vi "rt-Voltage - Continuous Output.vi"() -> ()   [LabVIEW 2019]
doc: "This example demonstrates how to continuously re-generate analog output data from a buffer in your computer's memory.\n\nRefer to your device documentation for pinouts and hardware capabilities."
uses:
  <vilib>/Utility/error.llb/DialogType.ctl
  <vilib>/DAQmx/write.llb/DAQmx Write (Analog 1D Wfm NChan NSamp).vi
  <vilib>/DAQmx/create/channels.llb/DAQmx Create Channel (AO-Voltage-Basic).vi
  <vilib>/DAQmx/configure/timing.llb/DAQmx Timing (Sample Clock).vi
  <vilib>/DAQmx/configure/trigger.llb/DAQmx Start Trigger (Digital Edge).vi
  <vilib>/DAQmx/configure/trigger.llb/DAQmx Start Trigger (Time).vi
  <vilib>/DAQmx/configure/trigger.llb/DAQmx Start Trigger (Analog Edge).vi
  <vilib>/DAQmx/miscellaneous.llb/DAQmx Fill In Error Info.vi
  <resource>/objmgr/daqmx.rc
  <vilib>/measure/NI_MABase.lvlib
panel:
  in  "Trigger Type":T1(tab)
  in  "Digital Start Trigger Edge":i32(ring)=10280 caption="Edge" items=["Rising"=10280, "Falling"=10171]
  in  "Digital Start Trigger Source":tag="/Dev1/PFI0" caption="Source"
  in  "Digital Pause Trigger Pause When":i32(ring)=10192 caption="Pause When" items=["High"=10192, "Low"=10214]
  in  "Digital Pause Trigger Source":tag="/Dev1/PFI0" caption="Source"
  in  "Analog Start Trigger Level":dbl caption="Level" format="%0.2f"
  in  "Analog Start Trigger Hysteresis":dbl caption="Hysteresis" format="%.2f"
  in  "Analog Start Trigger Slope":i32(ring)=10280 caption="Slope" items=["Rising"=10280, "Falling"=10171]
  in  "Analog Start Trigger Source":string="APFI0" caption="Source"
  in  "Analog Pause Trigger Source":string="APFI0" caption="Source"
  in  "Analog Pause Trigger Pause When":i32(ring)=10093 caption="Pause When" items=["Above Level"=10093, "Below Level"=10107]
  in  "Analog Pause Trigger Level":dbl caption="Level" format="%.2f"
  in  "When":timestamp
  in  "Select Time\nManually":bool
  in  "Output Array":T2(array[cluster])=[{"Waveform Type"=0, "Amplitude"=1.0, "Frequency"=10.0}] {"Frequency" format="%0.2p"; "Amplitude" format="%0.2p"; "Waveform Type" items=["Sine Wave", "Triangle Wave", "Square Wave", "Sawtooth Wave"]}
  in  "Number of Samples":i32=1000
  in  "Stop":bool
  out "Waveform Graph":waveform(dbl)[](graph)=[{"t0"=timestamp(0 s since 1904-01-01), "dt"=0.001, "Y"=[]}]
  in  "Sample Rate":dbl=1000.0
  in  "Sample Clock Source":tag="OnboardClock"
  in  "Max Voltage":dbl=5.0
  in  "Min Voltage":dbl=-5.0
  in  "Physical Channel(s)":tag="Dev1/ao0"
  out "Actual Sample Rate":dbl=1000.0 format="%0.2f"
  # "Channel Settings"
  # "Output"
  # "Timing and\nBuffer Settings"
  # "Waveform Settings"
  # "Trigger Settings"
  # "The number of elements in the waveform array must equal the number of channels in the task."
  # "To enable triggers, select a tab above, and configure the settings.\n\nNot all hardware supports all trigger types. Refer to your device documentation for more information."
  # "This trigger type is not supported in output tasks. \n\nRefer to your device documentation for more information on which triggers are supported."
  # "This trigger type is not supported in output tasks. \n\nRefer to your device documentation for more information on which triggers are supported."
  # "If time is not manually set, task will begin after 10 seconds"
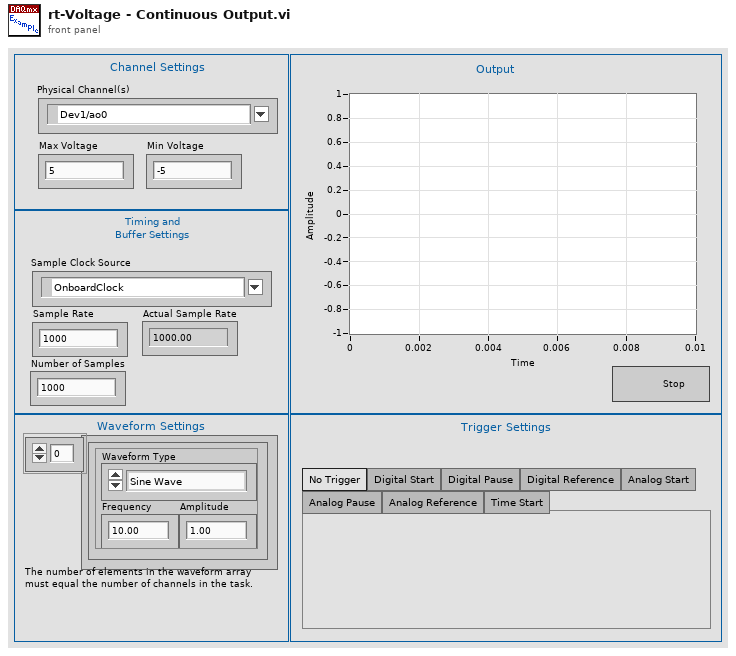
[diagram p1: front panel]
types:
  T1 = enum32{"No Trigger", "Digital Start", "Digital Pause", "Digital Reference", "Analog Start", "Analog Pause", "Analog Reference", "Time Start"}
  T2 = cluster{"Waveform Type":u16, "Amplitude":dbl, "Frequency":dbl}[]
  T3 = typedef "DialogType.ctl" = u16
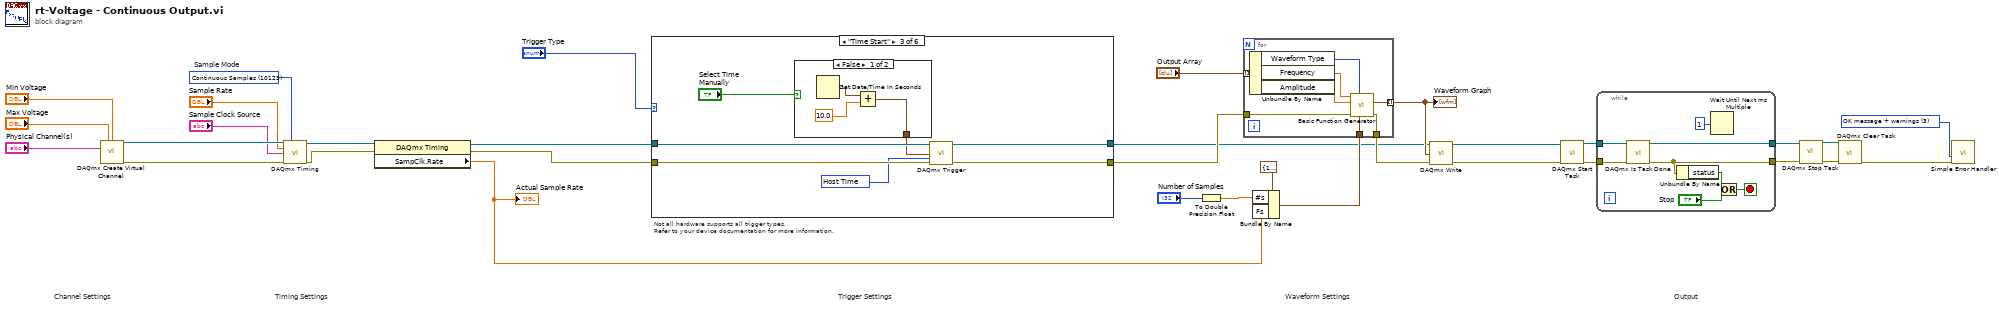
[diagram p0: block diagram]
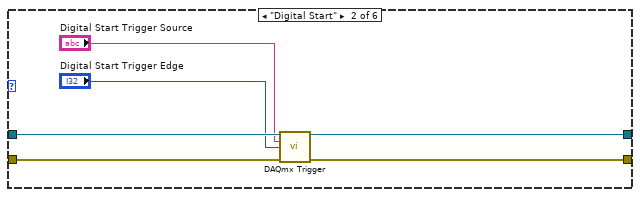
[diagram p3: hidden frame]
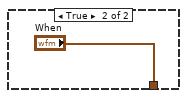
[diagram p4: hidden frame]
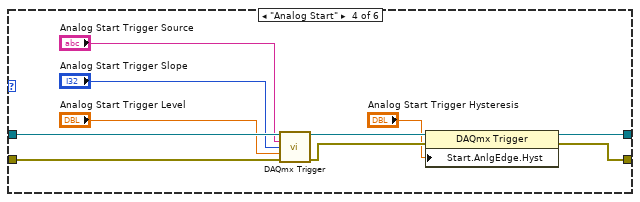
[diagram p5: hidden frame]
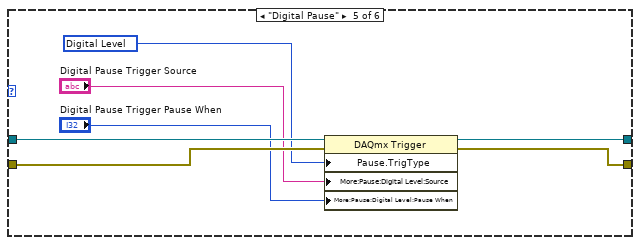
[diagram p6: hidden frame]
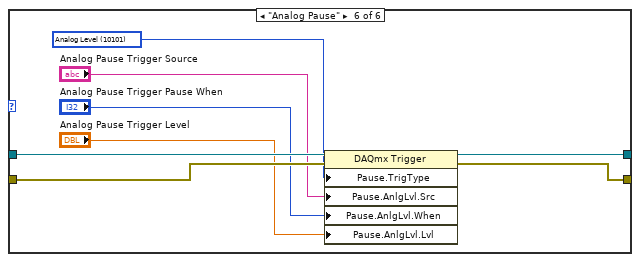
[diagram p7: hidden frame]
diagram:
  w6 = T3 3 items=["no dialog", "OK message", "continue or stop message", "OK message + warnings", "continue/stop + warnings"] ("type of dialog (OK msg:1)")
  w31 = 10123 items=["Finite Samples"=10178, "Continuous Samples"=10123, "Hardware Timed Single Point"=12522]  # Sample Mode
  # "Trigger Settings"
  # "Not all hardware supports all trigger types.\nRefer to your device documentation for more information."
  # "Output"
  # "Waveform Settings"
  # "Timing Settings"
  # "Channel Settings"
  n1 = call-poly <vilib>:"DAQmx Create Virtual Channel.vi"("maximum value"="Max Voltage", "minimum value"="Min Voltage", "physical channels"="Physical Channel(s)") -> ("task out"=w29:refnum<k21>, "error out"=w30:errorcluster)  [unwired: 11 in]
  n2 = call-poly <vilib>:"DAQmx Timing.vi"("task/channels in"=w29, "sample mode"=w31, "rate"="Sample Rate", "source"="Sample Clock Source", "error in"=w30) -> ("task out"=w33:refnum<k21>, "error out"=w32:errorcluster)  [unwired: 9 in]
  n3 = property class="DAQmx Timing"(reference=w33, error in=w32) -> (reference out=w4:refnum<k21>, error out=w3:errorcluster, "SampClk.Rate"=w19:dbl)
  "Actual Sample Rate" <- w19
  n4 = case shown="\"Time Start\"" "Trigger Type" {
    tunnel: w4 -> [w35 w41 w48 w62 w69 w77]
    tunnel: w3 -> [w34 w40 w47 w61 w66 w74]
    tunnel: [w35 w39 w46 w59 w68 w76] -> w1
    tunnel: [w34 w38 w45 w58 w67 w75] -> w2
    frame "No Trigger", Default {
    }
    frame "Digital Start" {
      n5 = call-poly <vilib>:"DAQmx Trigger.vi"("task/channels in"=w41, "source"="Digital Start Trigger Source", "edge"="Digital Start Trigger Edge", "error in"=w40) -> ("task out"=w39:refnum<k21>, "error out"=w38:errorcluster)  [unwired: 10 in]
    }
    frame "Time Start" {
      w44 = 16126 items=["Host Time"=16126, "I/O Device Time"=16127] ("timescale")
      n6 = case shown="False" "Select Time\nManually" {
        tunnel: [w50 "When"] -> w42
        frame False {
          n7 = Get Date/Time In Seconds() -> (seconds since 1Jan1904=w51:timestamp)
          n8 = Add(x=w51, y=10.0) -> (x+y=w50:timestamp)
        }
        frame True {
        }
      }
      n9 = call-poly <vilib>:"DAQmx Trigger.vi"("task/channels in"=w48, "when"=w42, "timescale"=w44, "error in"=w47) -> ("task out"=w46:refnum<k21>, "error out"=w45:errorcluster)  [unwired: 10 in]
    }
    frame "Analog Start" {
      n10 = call-poly <vilib>:"DAQmx Trigger.vi"("task/channels in"=w62, "source"="Analog Start Trigger Source", "slope"="Analog Start Trigger Slope", "level"="Analog Start Trigger Level", "error in"=w61) -> ("task out"=w57:refnum<k21>, "error out"=w56:errorcluster)  [unwired: 9 in]
      n11 = property class="DAQmx Trigger"(reference=w57, error in=w56, "Start.AnlgEdge.Hyst"="Analog Start Trigger Hysteresis") -> (reference out=w59:refnum<k21>, error out=w58:errorcluster)
    }
    frame "Digital Pause" {
      w65 = 10152 items=["Analog Level"=10101, "Analog Window"=10103, "Digital Level"=10152, "Digital Pattern"=10398, "None"=10230] ("Pause.TrigType")
      n12 = property class="DAQmx Trigger"(reference=w69, error in=w66, "Pause.TrigType"=w65, "More:Pause:Digital Level:Source"="Digital Pause Trigger Source", "More:Pause:Digital Level:Pause When"="Digital Pause Trigger Pause When") -> (reference out=w68:refnum<k21>, error out=w67:errorcluster)
    }
    frame "Analog Pause" {
      w73 = 10101 items=["Analog Level"=10101, "Analog Window"=10103, "Digital Level"=10152, "Digital Pattern"=10398, "None"=10230] ("Pause.TrigType")
      n13 = property class="DAQmx Trigger"(reference=w77, error in=w74, "Pause.TrigType"=w73, "Pause.AnlgLvl.Src"="Analog Pause Trigger Source", "Pause.AnlgLvl.When"="Analog Pause Trigger Pause When", "Pause.AnlgLvl.Lvl"="Analog Pause Trigger Level") -> (reference out=w76:refnum<k21>, error out=w75:errorcluster)
    }
  }
  n14 = To Double Precision Float(number="Number of Samples") -> (double precision float=w12:dbl)
  n15 = Bundle By Name(cluster=cluster{"Fs":dbl, "#s":dbl} {"Fs"=1000.0, "#s"=1000.0} ("sampling info"), "#s"=w12, "Fs"=w19) -> (w18:cluster{"Fs":dbl, "#s":dbl})
  n16 = for {
    tunnel: w2 -> [w85]
    tunnel: w18 -> [w84]
    tunnel: [w83] -> w15
    tunnel: "Output Array" -> [w82] mode=indexing
    tunnel: [w78] -> w13 mode=indexing
    n17 = Unbundle By Name(w82) -> ("Waveform Type"=w81:u16, "Frequency"=w80:dbl, "Amplitude"=w79:dbl)
    n18 = call <vilib>:"Basic Function Generator.vi"("sampling info"=w84, "signal type"=w81, "error in (no error)"=w85, "amplitude"=w79, "frequency"=w80) -> ("error out"=w83:errorcluster, "signal out"=w78:waveform(dbl))  [unwired: 4 in, 1 out]
  }
  "Waveform Graph" <- w13
  n19 = call-poly <vilib>:"DAQmx Write.vi"("task/channels in"=w1, "data"=w13, "error in"=w15) -> ("task out"=w17:refnum<k21>, "error out"=w16:errorcluster)  [unwired: 10 in, 1 out]
  n20 = call <vilib>:"DAQmx Start Task.vi"("task/channels in"=w17, "error in"=w16) -> ("task out"=w28:refnum<k21>, "error out"=w27:errorcluster)  [unwired: 12 in]
  n21 = while {
    tunnel: w28 -> [w93]
    tunnel: w27 -> [w92]
    tunnel: [w89] -> w7
    tunnel: [w90] -> w8
    stop <- w91 stop-if-true
    n22 = call <vilib>:"DAQmx Is Task Done.vi"("task/channels in"=w93, "error in"=w92) -> ("task out"=w90:refnum<k21>, "error out"=w89:errorcluster)  [unwired: 11 in, 1 out]
    n23 = Unbundle By Name(w89) -> ("status"=w88:bool)
    n24 = Wait Until Next ms Multiple(millisecond multiple=u32 1) -> ()  [unwired: 1 out]
    n25 = Or(x=w88, y="Stop") -> (x .or. y?=w91:bool)
  }
  n26 = call <vilib>:"DAQmx Stop Task.vi"("task/channels in"=w8, "error in"=w7) -> ("task out"=w10:refnum<k21>, "error out"=w9:errorcluster)  [unwired: 12 in]
  n27 = call <vilib>:"DAQmx Clear Task.vi"("task in"=w10, "error in"=w9) -> ("error out"=w26:errorcluster)  [unwired: 13 in]
  n28 = call <vilib>:"Simple Error Handler.vi"("type of dialog (OK msg:1)"=w6, "error in (no error)"=w26) -> ()  [unwired: 3 in, 5 out]
